vi "Day 17-Projectile Motion.vi"() -> ()   [LabVIEW 2021]
uses:
  1bdc6afe-5a0e-40ea-acba-09f2f6efd7f3.vi
  <vilib>/Utility/file.llb/Read Delimited Spreadsheet (I64).vi
  <vilib>/Comparison/Less/Less Functor/Less Functor.lvclass
panel:
  out "Possible Initial Velocities":cluster{i64, i64}[](array[cluster])
  out "Input":i64[](array[numeric])
  in  "Input File":enum32{"example input", "input"}(radio)
  out "Possibilities":i16
  out "Max y":i64
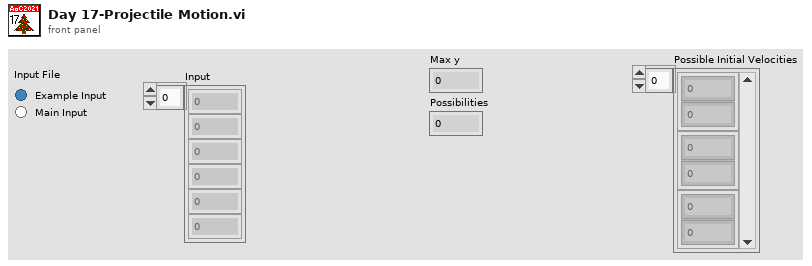
[diagram p1: front panel]
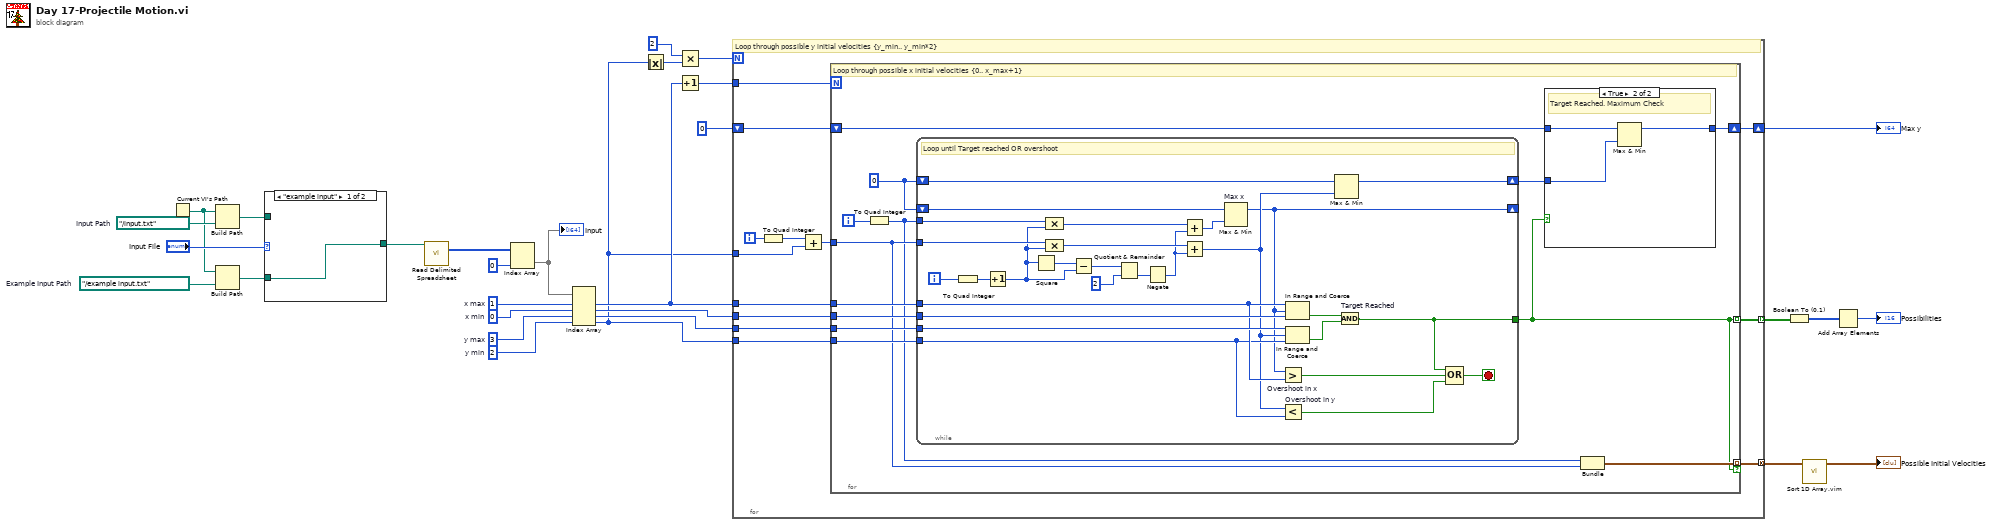
[diagram p0: block diagram]
diagram:
  w10 = 2  # y min
  w11 = 3  # y max
  w13 = 0  # x min
  w14 = 1  # x max
  w23 = path "../example input.txt"  # Example Input Path
  w24 = path "../input.txt"  # Input Path
  n1 = Current VI's Path() -> (path=w18:path)
  n2 = Build Path(base path=w18, name or relative path=w24) -> (appended path=w21:path)
  n3 = Build Path(base path=w18, name or relative path=w23) -> (appended path=w20:path)
  n4 = case shown="\"example input\"" "Input File" {
    tunnel: w21 -> [_ w31]
    tunnel: w20 -> [w30 _]
    tunnel: [w30 w31] -> w19
    frame "example input" {
    }
    frame "input" {
    }
  }
  n5 = call-poly <vilib>:"Read Delimited Spreadsheet.vi"("file path (dialog if empty)"=w19) -> ("all rows"=w17:i64[][])  [unwired: 9 in, 5 out]
  n6 = Index Array(array=w17, index (col)=0 ("disabled index (col)")) -> (element=w15:i64[])  [unwired: 1 in]
  "Input" <- w15
  n7 = Index Array(array=w15, index #1=w14, index #2=w13, index #3=w11, index #4=w10) -> (element #1=w8:i64, element #2=w12:i64, element #3=w9:i64, element #4=w3:i64)
  n8 = Absolute Value(x=w3) -> (abs(x)=w6:i64)
  n9 = Multiply(x=i64 2, y=w6) -> (x*y=w4:i64)
  n10 = Increment(x=w8) -> (x+1=w7:i64)
  n11 = for {
    N: w4 -> [_]
    tunnel: w8 -> [w44]
    tunnel: w12 -> [w43]
    tunnel: w9 -> [w42]
    tunnel: w3 -> [w41]
    shift-right: [w39] -> w28
    shift-left: i64 0 -> [w40]
    tunnel: [w38] -> w27 mode=indexing
    tunnel: w3 -> [w36]
    tunnel: w7 -> [w34]
    tunnel: [w33] -> w2 mode=concatenating
    i -> [w37]
    # "Loop through possible y initial velocities {y_min.. y_min*2}"
    n12 = To Quad Integer(1:w37) -> (0:w35:i64)
    n13 = Add(x=w35, y=w36) -> (x+y=w32:i64)
    n14 = for {
      N: w34 -> [_]
      tunnel: w32 -> [w49]
      tunnel: w44 -> [w57]
      tunnel: w43 -> [w56]
      tunnel: w42 -> [w55]
      tunnel: w41 -> [w54]
      shift-right: [w51] -> w39
      shift-left: w40 -> [w53]
      tunnel: [w47] -> w38 mode=indexing
      tunnel: [w48] -> w33 mode=indexing if=w47
      i -> [w50]
      w46 = i64 0
      # "Loop through possible x initial velocities {0.. x_max+1}"
      n15 = To Quad Integer(1:w50) -> (0:w45:i64)
      n16 = while {
        tunnel: w57 -> [w79]
        tunnel: w56 -> [w83]
        tunnel: w55 -> [w81]
        tunnel: w54 -> [w74]
        shift-right: [w76] -> w52
        shift-left: w46 -> [w75]
        tunnel: [w73] -> w47
        tunnel: w45 -> [w85]
        tunnel: w49 -> [w67]
        shift-right: [w59] -> _
        shift-left: w46 -> [w60]
        i -> [w72]
        stop <- w84 stop-if-true
        # "Loop until Target reached OR overshoot"
        n17 = To Quad Integer(1:w72) -> (0:w64:i64)
        n18 = Increment(x=w64) -> (x+1=w63:i64)
        n19 = Square(x=w63) -> (x^2=w71:i64)
        n20 = Compound Arithmetic op=MULTIPLY(w85, w63) -> (w61:i64)
        n21 = Compound Arithmetic op=MULTIPLY(w67, w63) -> (w66:i64)
        n22 = Subtract(x=w71, y=w63) -> (x-y=w70:i64)
        n23 = Quotient & Remainder(x=w70, y=i64 2) -> (floor(x/y)=w68:i64)  [unwired: 1 out]
        n24 = Negate(x=w68) -> (-x=w62:i64)
        n25 = Add(x=w61, y=w62) -> (x+y=w58:i64)
        n26 = Add(x=w66, y=w62) -> (x+y=w65:i64)
        n27 = Max & Min "Max x"(x=w60, y=w58) -> (max(x,y)=w59:i64)  [unwired: 1 out]
        n28 = Greater? "Overshoot in x"(x=w59, y=w79) -> (0:w78:bool)
        n29 = Less? "Overshoot in y"(x=w65, y=w74) -> (x < y?=w77:bool)
        n30 = In Range and Coerce(upper limit=w79, x=w59, lower limit=w83) -> (In Range?=w82:bool)  [unwired: 1 out]
        n31 = In Range and Coerce(upper limit=w81, x=w65, lower limit=w74) -> (In Range?=w80:bool)  [unwired: 1 out]
        n32 = Max & Min(x=w75, y=w65) -> (max(x,y)=w76:i64)  [unwired: 1 out]
        n33 = Compound Arithmetic op=AND "Target Reached"(w82, w80) -> (w73:bool)
        n34 = Compound Arithmetic op=OR(w73, w78, w77) -> (w84:bool)
      }
      n35 = case shown="True" w47 {
        tunnel: w53 -> [w86 w89]
        tunnel: w52 -> [_ w88]
        tunnel: [w86 w87] -> w51
        frame False {
          # "Target not Reached"
        }
        frame True {
          # "Target Reached. Maximum Check"
          n36 = Max & Min(x=w89, y=w88) -> (max(x,y)=w87:i64)  [unwired: 1 out]
        }
      }
      n37 = Bundle(w45, w49) -> (w48:cluster{i64, i64})  [unwired: 1 in]
    }
  }
  "Max y" <- w28
  n38 = Boolean To (0,1)(Boolean=w27) -> (0, 1=w26:i16[][])
  n39 = call "Sort 1D Array.vim"("unsorted array"=w2) -> ("sorted array"=→"Possible Initial Velocities":cluster{i64, i64}[])  [unwired: 10 in]
  n40 = Add Array Elements(numeric array=w26) -> (sum=→"Possibilities":i16)
